vi "fisiere_v3.vi"() -> ()   [LabVIEW 2009]
panel:
  out "Nr_i":dbl
  out "Citire din fisier terminata":bool
  in  "Selectati calea si fisierul":path=path "E:/Projects/Lab_view/Vi/fisiere/country-capital.txt"
  # "Numarul de inregistrari gasite"
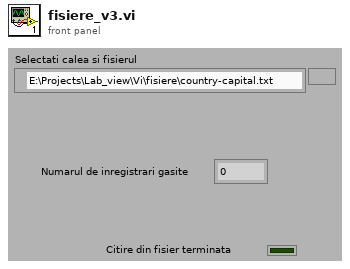
[diagram p1: front panel]
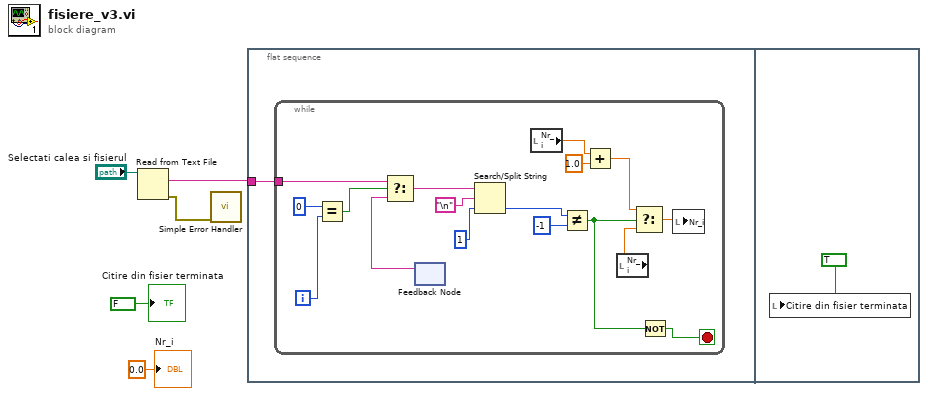
[diagram p0: block diagram]
diagram:
  n1 = Read from Text File(file (use dialog)="Selectati calea si fisierul") -> (text=w4:string, error out=w3:errorcluster)  [unwired: 3 in, 2 out]
  n2 = call <vilib>:"Simple Error Handler.vi"("error in (no error)"=w3) -> ()  [unwired: 4 in, 5 out]
  n3 = flat-sequence {
    tunnel: w4 -> [w6]
    frame #0 {
      n4 = while {
        tunnel: w6 -> [w21]
        i -> [w20]
        stop <- w7 stop-if-true
        n5 = Equal?(x=0, y=w20) -> (x = y?=w18:bool)
        n6 = feedback #1() -> (w22:string)  [unwired: 1 in]
        n7 = Select(t=w21, s=w18, f=w22) -> (s? t:f=w17:string)
        n8 = Search/Split String(string=w17, search string/char (-)="\n", offset (0)=1) -> (match + rest of string=w16:string, offset of match=w11:i32)  [unwired: 1 out]
        n9 = local read "Nr_i"() -> (w14:dbl)
        n10 = Not Equal?(x=w11, y=-1) -> (x != y?=w8:bool)
        n11 = Add(x=w14, y=1.0) -> (x+y=w13:dbl)
        n12 = local read "Nr_i"() -> (w9:dbl)
        n13 = Select(t=w13, s=w8, f=w9) -> (s? t:f=w12:dbl)
        n14 = Not(x=w8) -> (.not. x?=w7:bool)
        n15 = local write "Nr_i"(w12) -> ()
      }
    }
    frame #1 {
      n16 = local write "Citire din fisier terminata"(TRUE ("Ready")) -> ()
    }
  }
  "Citire din fisier terminata" <- FALSE ("Af_start")
  "Nr_i" <- 0.0 ("Nr_i")
